vi "SwitchOrKeep.vi"(10 "Rising flank? in":bool, 11 "Last state in":bool) -> (3 "New state out":bool)   [LabVIEW 2012]
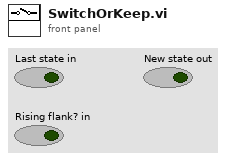
[diagram p1: front panel]
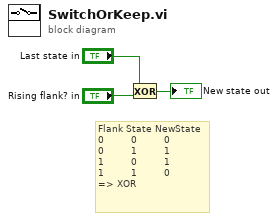
[diagram p0: block diagram]
diagram:
  # "Flank State NewState\n0         0         0\n0         1         1\n1         0         1\n1         1         0\n=> XOR"
  n1 = Exclusive Or(1:"Rising flank? in", 2:"Last state in") -> (0:→"New state out":bool)
